vi "Sabertooths in use FGV wrapper.vi"(8 "error in (no error)":errorcluster) -> (0 "error out":errorcluster)   [LabVIEW 2018]
uses:
  controls/Sabertooth Address Select.ctl
  Sabertooths in use gvar.vi
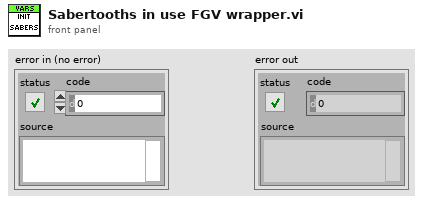
[diagram p1: front panel]
types:
  T1 = typedef "Sabertooth Address Select.ctl" = u8
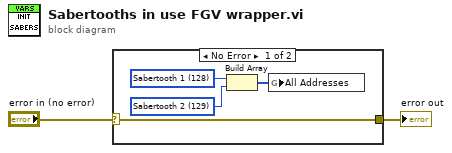
[diagram p0: block diagram]
diagram:
  n1 = case shown="No Error" "error in (no error)" {
    selector: "error in (no error)" -> [w3 w7]
    tunnel: [w3 w7] -> w1
    frame No Error {
      w5 = T1 128 items=["Sabertooth 1"=128, "Sabertooth 2"=129, "Sabertooth 3"=130, "Sabertooth 4"=131, "Sabertooth 5"=132, "Sabertooth 6"=133, "Sabertooth 7"=134, "Sabertooth 8"=135] ("Sabertooth Addresses")
      w6 = T1 129 items=["Sabertooth 1"=128, "Sabertooth 2"=129, "Sabertooth 3"=130, "Sabertooth 4"=131, "Sabertooth 5"=132, "Sabertooth 6"=133, "Sabertooth 7"=134, "Sabertooth 8"=135] ("Sabertooth Addresses")
      n2 = Build Array(w5, w6) -> (w4:T1[])
      n3 = global write "Sabertooths in use gvar.vi" "All Addresses"(w4) -> ()
    }
    frame Error {
    }
  }
  "error out" <- w1
